vi "AP2x4x SelectResolutionFreq.vi"(7 "Resolution":enum16{"5MHz", "180MHz"}(ring), 8 "error in":errorcluster, 11 "AP2x4x IN":refnum<visa-resource-name>="TCPIP0::169.254.53.138::5900::SOCKET") -> (0 "error out":errorcluster, 3 "AP2x4x OUT":refnum<visa-resource-name>="TCPIP0::169.254.53.138::5900::SOCKET")   [LabVIEW 2014]
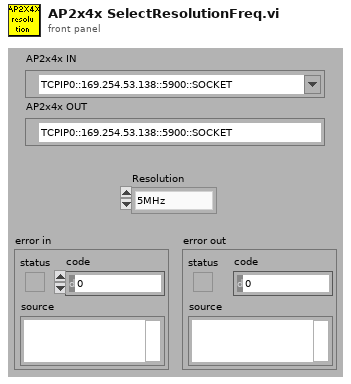
[diagram p1: front panel]
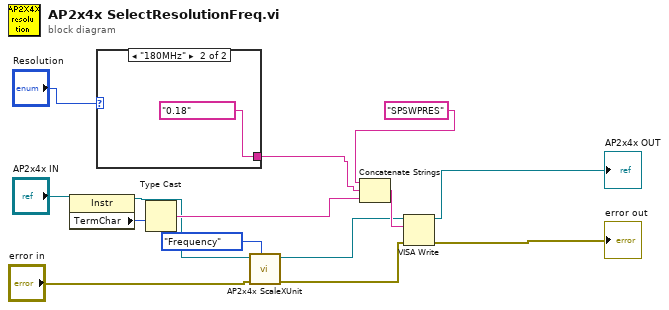
[diagram p0: block diagram]
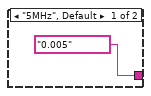
[diagram p2: hidden frame]
diagram:
  n1 = property class="Instr"(reference="AP2x4x IN") -> (reference out=w5:refnum<visa-resource-name>, "TermChar"=w6:u8)  [unwired: 1 in, 1 out]
  n2 = case shown="\"180MHz\"" "Resolution" {
    tunnel: ["0.005" "0.18"] -> w7
    frame "5MHz", Default {
    }
    frame "180MHz" {
    }
  }
  n3 = Type Cast(x=w6) -> (*(type *) &x=w9:string)  [unwired: 1 in]
  n4 = call "AP2x4x ScaleXUnit.vi"("Unit"=enum16{"Frequency", "Wavelength"}."Frequency", "error in"="error in", "AP2x4x IN"=w5) -> ("error out"=w3:errorcluster, "AP2x4x OUT"=w2:refnum<visa-resource-name>)  [unwired: 7 in]
  n5 = Concatenate Strings("SPSWPRES" ("data string"), w7, w9) -> (w14:string)
  n6 = VISA Write(VISA resource name=w2, write buffer=w14, error in (no error)=w3) -> (VISA resource name out=→"AP2x4x OUT":refnum<visa-resource-name>, error out=→"error out":errorcluster)  [unwired: 1 out]
